vi "Amplifier Daemon.vi"(0 "Multiclamp Reference":i32, 1 "Signal":refnum<vi>, 2 "Gain":refnum<vi>, 3 "Autotune Gain":T4, 4 "Test Signal":T3, 5 "Error In":errorcluster, 6 "Capacitance Compensation":T5, 7 "Pipette Offset":T1, 9 "Holding Potential":T2, 11 "Reset":refnum<vi>, 13 "Exit":refnum<vi>) -> (19 "Error Out":errorcluster)   [LabVIEW 2012, in "MultiClamp 700B Controls.lvlib"]
uses:
  MultiClamp 700B Controls.lvlib
  AxMultiClampMsg/AxMultiClampMsg.lvlib
panel:
  out "Exit":bool
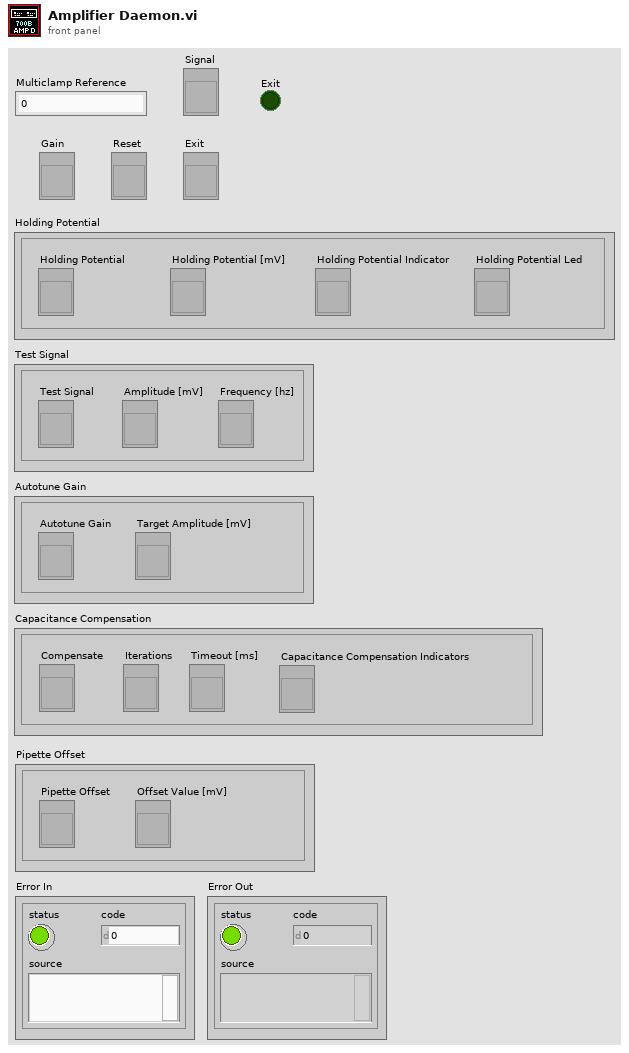
[diagram p1: front panel]
types:
  T1 = cluster{"Pipette Offset":refnum<vi>, "Offset Value [mV]":refnum<vi>}
  T2 = cluster{"Holding Potential [mV]":refnum<vi>, "Holding Potential":refnum<vi>, "Holding Potential Indicator":refnum<vi>, "Holding Potential Led":refnum<vi>}
  T3 = cluster{"Test Signal":refnum<vi>, "Amplitude [mV]":refnum<vi>, "Frequency [hz]":refnum<vi>}
  T4 = cluster{"Autotune Gain":refnum<vi>, "Target Amplitude [mV]":refnum<vi>}
  T5 = cluster{"Timeout [ms]":refnum<vi>, "Iterations":refnum<vi>, "Compensate":refnum<vi>, "Capacitance Compensation Indicators":refnum<vi>}
  T6 = cluster{"Cp Fast [pF]":dbl, "Cp Slow [pF]":dbl, "Tau Fast [um]":dbl, "Tau Slow [um]":dbl}
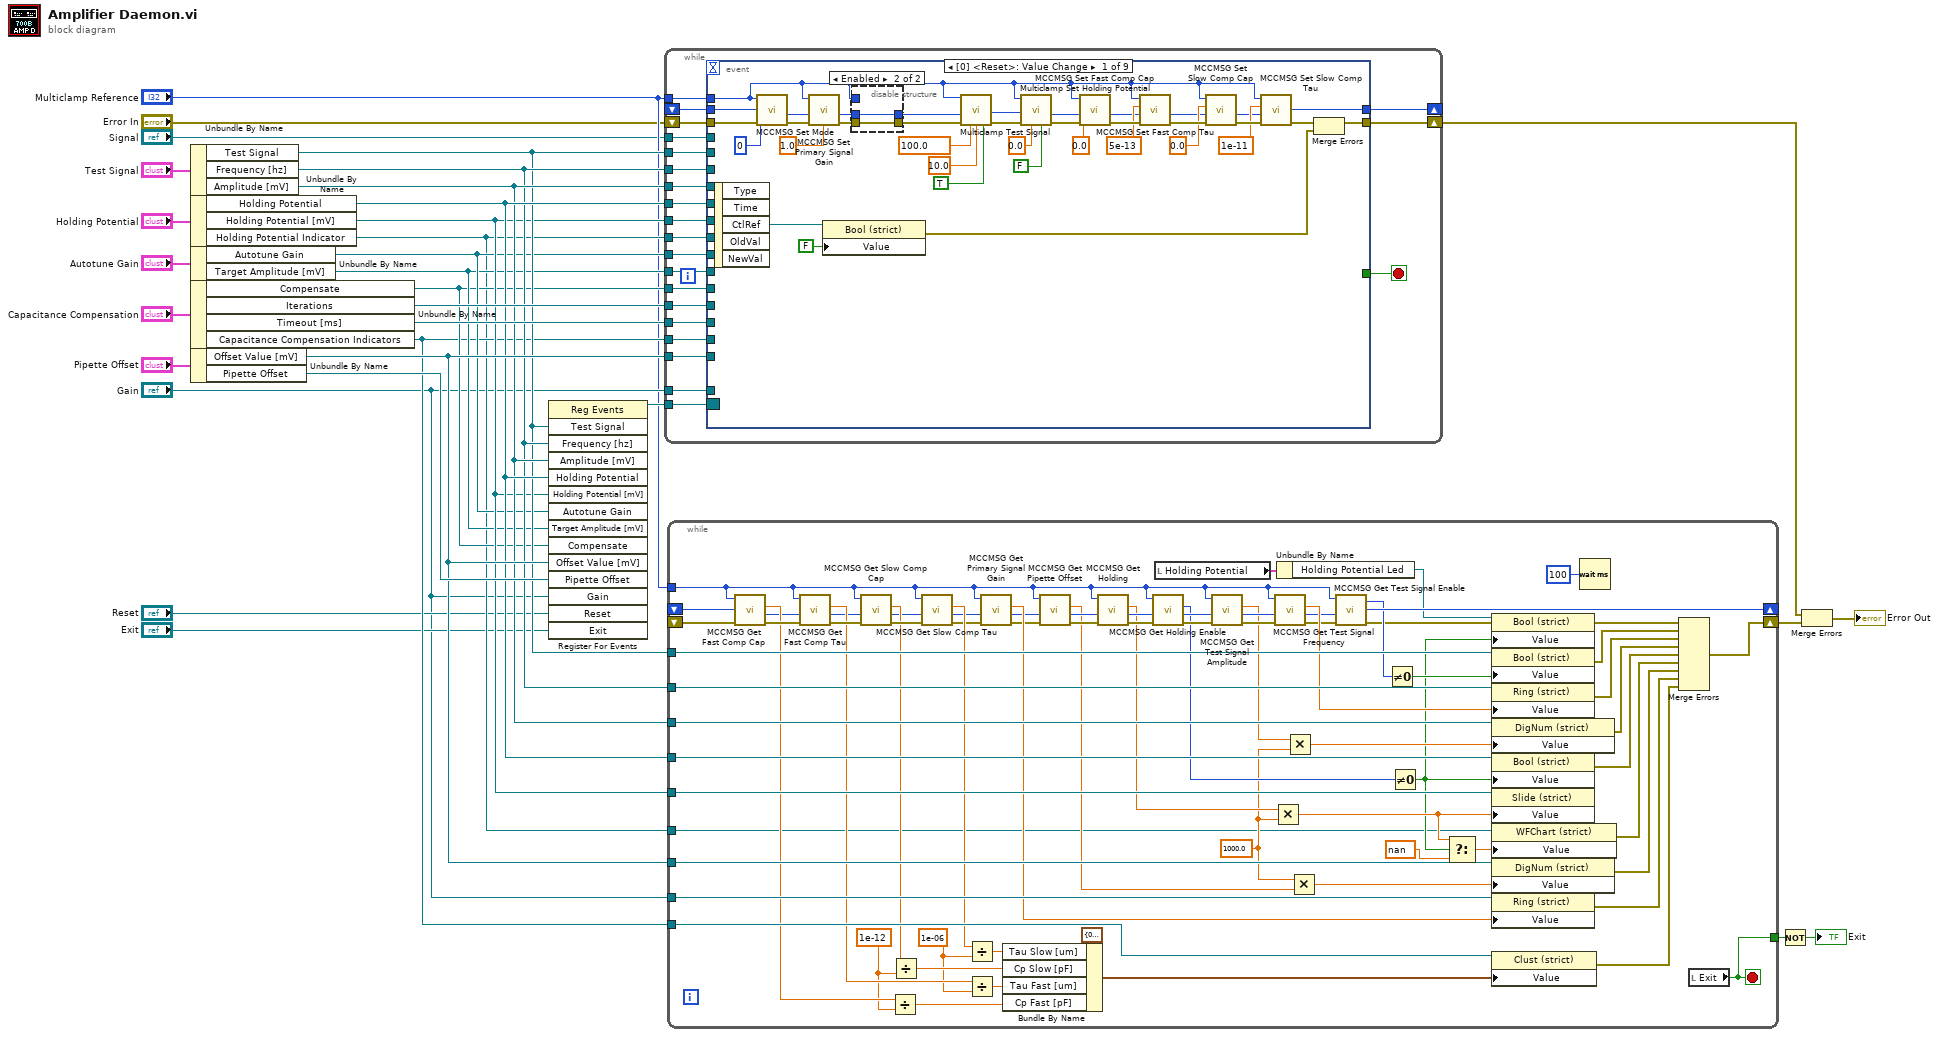
[diagram p0: block diagram]
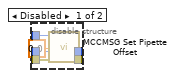
[diagram p2: hidden frame]
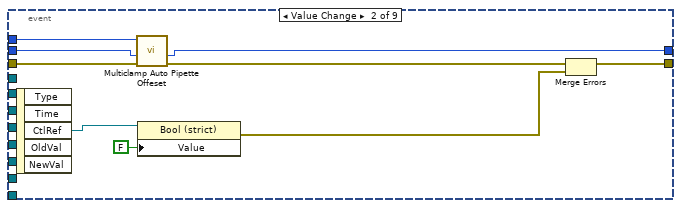
[diagram p3: hidden frame]
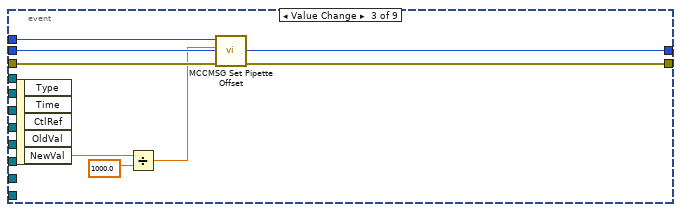
[diagram p4: hidden frame]
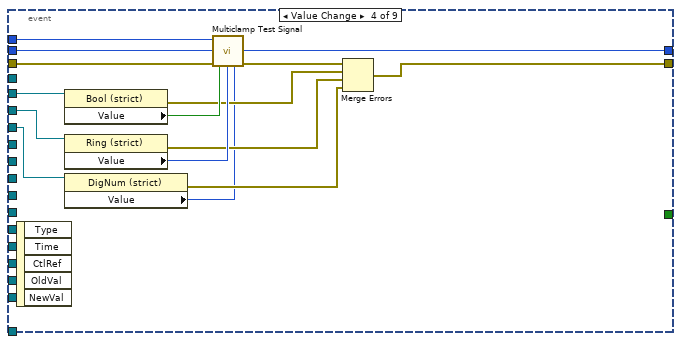
[diagram p5: hidden frame]
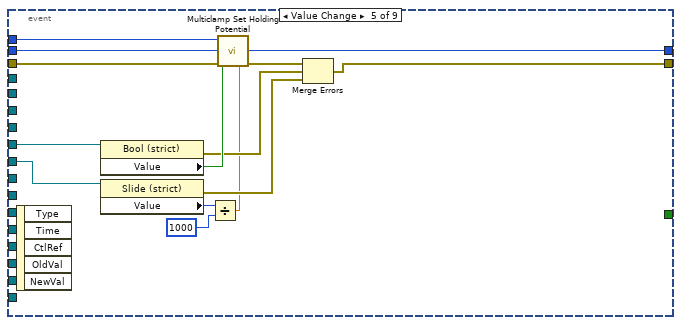
[diagram p6: hidden frame]
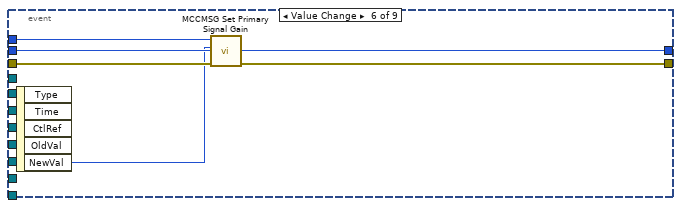
[diagram p7: hidden frame]
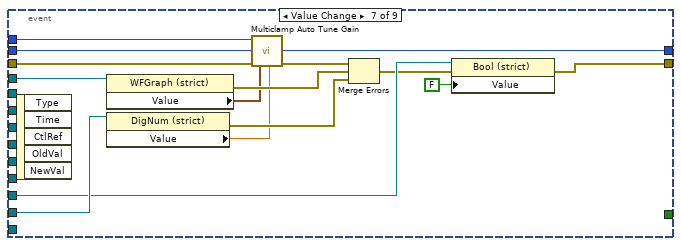
[diagram p8: hidden frame]
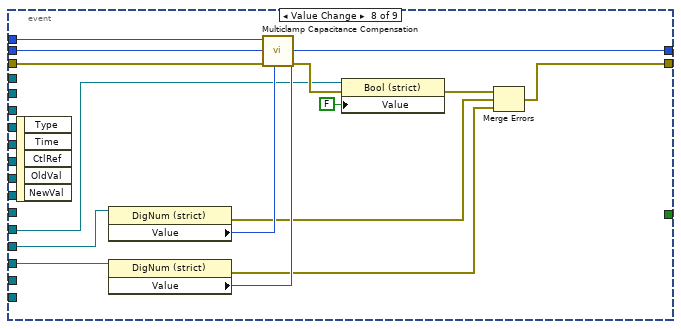
[diagram p9: hidden frame]
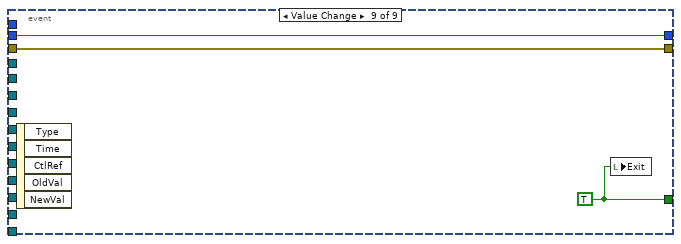
[diagram p10: hidden frame]
diagram:
  n1 = Unbundle By Name("Test Signal") -> ("Test Signal"=w23:refnum<vi>, "Frequency [hz]"=w24:refnum<vi>, "Amplitude [mV]"=w25:refnum<vi>)
  n2 = Unbundle By Name("Holding Potential") -> ("Holding Potential"=w26:refnum<vi>, "Holding Potential [mV]"=w22:refnum<vi>, "Holding Potential Indicator"=w17:refnum<vi>)
  n3 = Unbundle By Name("Autotune Gain") -> ("Autotune Gain"=w21:refnum<vi>, "Target Amplitude [mV]"=w20:refnum<vi>)
  n4 = Unbundle By Name("Capacitance Compensation") -> ("Compensate"=w19:refnum<vi>, "Iterations"=w30:refnum<vi>, "Timeout [ms]"=w29:refnum<vi>, "Capacitance Compensation Indicators"=w18:refnum<vi>)
  n5 = Unbundle By Name("Pipette Offset") -> ("Offset Value [mV]"=w27:refnum<vi>, "Pipette Offset"=w28:refnum<vi>)
  n6 = register-events(w23, w24, w25, w26, w22, w21, w20, w19, w27, w28, "Gain", "Reset", "Exit") -> (reference out=w31:refnum<event-registration>)  [unwired: 2 in, 1 out]
  n7 = while {
    tunnel: w31 -> [w53]
    tunnel: "Multiclamp Reference" -> [w52]
    tunnel: w24 -> [w51]
    tunnel: w25 -> [w50]
    tunnel: w23 -> [w49]
    tunnel: w26 -> [w48]
    tunnel: w22 -> [w47]
    tunnel: w20 -> [w46]
    tunnel: "Signal" -> [w45]
    tunnel: w30 -> [w44]
    tunnel: w29 -> [w43]
    tunnel: w21 -> [w42]
    tunnel: w19 -> [w41]
    shift-right: [w40] -> w15
    shift-left: "Error In" -> [w39]
    tunnel: w27 -> [w38]
    shift-right: [w36] -> _
    shift-left: _ -> [w37]
    tunnel: w18 -> [w34]
    tunnel: w17 -> [w33]
    tunnel: "Gain" -> [w32]
    stop <- w35 stop-if-true
    n8 = event shown="[0] <Reset>: Value Change" {
      selector: w53 -> [_ _ _ _ _ _ _ _ _]
      dyn-events: _ -> [_ _ _ _ _ _ _ _ _]
      timeout: _ -> [_ _ _ _ _ _ _ _ _]
      tunnel: w52 -> [w75 w106 w114 w129 w141 w148 w163 w179 _]
      tunnel: w51 -> [_ _ _ w128 _ _ _ _ _]
      tunnel: w50 -> [_ _ _ w116 _ _ _ _ _]
      tunnel: w49 -> [_ _ _ w126 _ _ _ _ _]
      tunnel: w48 -> [_ _ _ _ w143 _ _ _ _]
      tunnel: w47 -> [_ _ _ _ w142 _ _ _ _]
      tunnel: w46 -> [_ _ _ _ _ _ w164 _ _]
      tunnel: w45 -> [_ _ _ _ _ _ w162 _ _]
      tunnel: w44 -> [_ _ _ _ _ _ _ w176 _]
      tunnel: w43 -> [_ _ _ _ _ _ _ w177 _]
      tunnel: w42 -> [_ _ _ _ _ _ w161 _ _]
      tunnel: w41 -> [_ _ _ _ _ _ _ w166 _]
      tunnel: [w67 w100 w112 w119 w135 w147 w152 w172 w181] -> w40
      tunnel: w39 -> [w77 w104 w113 w124 w139 w149 w159 w174 w181]
      tunnel: w38 -> [_ _ _ _ _ _ _ _ _]
      tunnel: w37 -> [w64 w102 w111 w118 w134 w145 w156 w168 w182]
      tunnel: [w55 w101 w110 w117 w133 w146 w155 w167 w182] -> w36
      tunnel: [_ _ _ _ _ _ _ _ w180] -> w35
      tunnel: w34 -> [_ _ _ _ _ _ _ _ _]
      tunnel: w33 -> [_ _ _ _ _ _ _ _ _]
      tunnel: w32 -> [_ _ _ _ _ _ _ _ _]
      event Value Change {
        w73 = 100.0 items=["2 Hz"=2.0, "5 Hz"=5.0, "10 Hz"=10.0, "20 Hz"=20.0, "50 Hz"=50.0, "60 Hz"=60.0, "100 Hz"=100.0, "200 Hz"=200.0, "500 Hz"=500.0, "1000 Hz"=1000.0] ("Frequency")
        n9 = event-data() -> ("CtlRef"=w68:refnum<vi>)  [unwired: 1 in, 4 out]
        n10 = call "MCCMSG Set Mode.vi"("error in (no error)"=w77, "pnError"=w64, "uModeID"=u32 0, "hMCCmsg"=w75) -> ("error out"=w76:errorcluster, "pnError out"=w63:i32)  [unwired: 5 in, 1 out]
        n11 = call "MCCMSG Set Primary Signal Gain.vi"("error in (no error)"=w76, "pnError"=w63, "dGain"=1.0, "hMCCmsg"=w75) -> ("error out"=w89:errorcluster, "pnError out"=w62:i32)  [unwired: 5 in, 1 out]
        n12 = property class="Bool (strict)"(reference=w68, "Value"=FALSE) -> (error out=w65:errorcluster)  [unwired: 1 in, 1 out]
        n13 = disable-structure shown="Enabled" {
          disable-tunnel: w89 -> [w95 w97]
          disable-tunnel: [w94 w97] -> w80
          disable-tunnel: w75 -> [w93 _]
          disable-tunnel: w62 -> [w92 w96]
          disable-tunnel: [w91 w96] -> w61
          frame Disabled {
            n14 = call "MCCMSG Set Pipette Offset.vi"("error in (no error)"=w95, "pnError"=w92, "dPipetteOffset"=0.0, "hMCCmsg"=w93) -> ("error out"=w94:errorcluster, "pnError out"=w91:i32)  [unwired: 5 in, 1 out]
          }
          frame Enabled {
          }
        }
        n15 = call "Multiclamp Test Signal.vi"("Handler"=w75, "set"=TRUE, "pnErrorIn"=w61, "error in (no error)"=w80, "Frequency"=w73, "Amplitude [mV]"=10.0 ("Amplitude")) -> ("pnError out"=w60:i32, "error out"=w79:errorcluster)  [unwired: 7 in, 1 out]
        n16 = call "Multiclamp Set Holding Potential.vi"("On"=FALSE, "error in (no error)"=w79, "Voltage"=0.0, "pnError"=w60, "hMCCmsg"=w75) -> ("error out"=w78:errorcluster, "pnError out"=w56:i32)  [unwired: 4 in, 1 out]
        n17 = call "MCCMSG Set Fast Comp Cap.vi"("error in (no error)"=w78, "pnError"=w56, "dFastCompCap"=0.0, "hMCCmsg"=w75) -> ("error out"=w88:errorcluster, "pnError out"=w57:i32)  [unwired: 5 in, 1 out]
        n18 = call "MCCMSG Set Fast Comp Tau.vi"("error in (no error)"=w88, "pnError"=w57, "dFastCompTau"=5e-13, "hMCCmsg"=w75) -> ("error out"=w87:errorcluster, "pnError out"=w58:i32)  [unwired: 5 in, 1 out]
        n19 = call "MCCMSG Set Slow Comp Cap.vi"("error in (no error)"=w87, "pnError"=w58, "dSlowCompCap"=0.0, "hMCCmsg"=w75) -> ("error out"=w86:errorcluster, "pnError out"=w59:i32)  [unwired: 5 in, 1 out]
        n20 = call "MCCMSG Set Slow Comp Tau.vi"("error in (no error)"=w86, "pnError"=w59, "dSlowCompTau"=1e-11, "hMCCmsg"=w75) -> ("error out"=w66:errorcluster, "pnError out"=w55:i32)  [unwired: 5 in, 1 out]
        n21 = Merge Errors(w66, w65) -> (w67:errorcluster)
      }
      event Value Change {
        n22 = event-data() -> ("CtlRef"=w105:refnum<vi>)  [unwired: 1 in, 4 out]
        n23 = call "Multiclamp Auto Pipette Offeset.vi"("error in (no error)"=w104, "pnError"=w102, "hMCCmsg"=w106) -> ("error out"=w103:errorcluster, "pnError out"=w101:i32)  [unwired: 6 in, 1 out]
        n24 = property class="Bool (strict)"(reference=w105, "Value"=FALSE) -> (error out=w99:errorcluster)  [unwired: 1 in, 1 out]
        n25 = Merge Errors(w103, w99) -> (w100:errorcluster)
      }
      event Value Change {
        n26 = event-data() -> ("NewVal"=w109:dbl)  [unwired: 1 in, 4 out]
        n27 = Divide(x=w109, y=1000.0) -> (x/y=w108:dbl)
        n28 = call "MCCMSG Set Pipette Offset.vi"("error in (no error)"=w113, "pnError"=w111, "dPipetteOffset"=w108, "hMCCmsg"=w114) -> ("error out"=w112:errorcluster, "pnError out"=w110:i32)  [unwired: 5 in, 1 out]
      }
      event Value Change {
        n29 = event-data() -> ()  [unwired: 1 in, 5 out]
        n30 = property class="Bool (strict)"(reference=w126) -> (error out=w122:errorcluster, "Value"=w127:bool)  [unwired: 1 in, 1 out]
        n31 = property class="Ring (strict)"(reference=w128) -> (error out=w121:errorcluster, "Value"=w125:u16)  [unwired: 1 in, 1 out]
        n32 = property class="DigNum (strict)"(reference=w116) -> (error out=w120:errorcluster, "Value"=w115:i32)  [unwired: 1 in, 1 out]
        n33 = call "Multiclamp Test Signal.vi"("Handler"=w129, "set"=w127, "pnErrorIn"=w118, "error in (no error)"=w124, "Frequency"=w125, "Amplitude [mV]"=w115) -> ("pnError out"=w117:i32, "error out"=w123:errorcluster)  [unwired: 7 in, 1 out]
        n34 = Merge Errors(w123, w122, w121, w120) -> (w119:errorcluster)
      }
      event Value Change {
        n35 = event-data() -> ()  [unwired: 1 in, 5 out]
        n36 = property class="Bool (strict)"(reference=w143) -> (error out=w137:errorcluster, "Value"=w140:bool)  [unwired: 1 in, 1 out]
        n37 = property class="Slide (strict)"(reference=w142) -> (error out=w136:errorcluster, "Value"=w132:i32)  [unwired: 1 in, 1 out]
        n38 = Divide(x=w132, y=1000) -> (x/y=w131:dbl)
        n39 = call "Multiclamp Set Holding Potential.vi"("On"=w140, "error in (no error)"=w139, "Voltage"=w131, "pnError"=w134, "hMCCmsg"=w141) -> ("error out"=w138:errorcluster, "pnError out"=w133:i32)  [unwired: 4 in, 1 out]
        n40 = Merge Errors(w138, w137, w136) -> (w135:errorcluster)
      }
      event Value Change {
        n41 = event-data() -> ("NewVal"=w144:u16)  [unwired: 1 in, 4 out]
        n42 = call "MCCMSG Set Primary Signal Gain.vi"("error in (no error)"=w149, "pnError"=w145, "dGain"=w144, "hMCCmsg"=w148) -> ("error out"=w147:errorcluster, "pnError out"=w146:i32)  [unwired: 5 in, 1 out]
      }
      event Value Change {
        n43 = event-data() -> ()  [unwired: 1 in, 5 out]
        n44 = property class="WFGraph (strict)"(reference=w162) -> (error out=w157:errorcluster, "Value"=w151:waveform(dbl))  [unwired: 1 in, 1 out]
        n45 = property class="DigNum (strict)"(reference=w164) -> (error out=w154:errorcluster, "Value"=w150:dbl)  [unwired: 1 in, 1 out]
        n46 = call "Multiclamp Auto Tune Gain.vi"("Target Delta pp"=w150, "error in (no error)"=w159, "pnError"=w156, "Multiclamp Reference"=w163, "Test Signal"=w151) -> ("error out"=w158:errorcluster, "pnError out"=w155:i32)  [unwired: 3 in, 2 out]
        n47 = Merge Errors(w158, w157, w154) -> (w153:errorcluster)
        n48 = property class="Bool (strict)"(reference=w161, error in=w153, "Value"=FALSE) -> (error out=w152:errorcluster)  [unwired: 1 out]
      }
      event Value Change {
        n49 = event-data() -> ()  [unwired: 1 in, 5 out]
        n50 = property class="DigNum (strict)"(reference=w176) -> (error out=w170:errorcluster, "Value"=w175:i32)  [unwired: 1 in, 1 out]
        n51 = property class="DigNum (strict)"(reference=w177) -> (error out=w169:errorcluster, "Value"=w178:u32)  [unwired: 1 in, 1 out]
        n52 = call "Multiclamp Capacitance Compensation.vi"("#i"=w175, "error in (no error)"=w174, "Timeout [ms]"=w178, "pnError"=w168, "hMCCmsg"=w179) -> ("error out"=w173:errorcluster, "pnError out"=w167:i32)  [unwired: 4 in, 1 out]
        n53 = property class="Bool (strict)"(reference=w166, error in=w173, "Value"=FALSE) -> (error out=w171:errorcluster)  [unwired: 1 out]
        n54 = Merge Errors(w171, w170, w169) -> (w172:errorcluster)
      }
      event Value Change {
        w180 = TRUE ("NewVal")
        n55 = event-data() -> ()  [unwired: 1 in, 5 out]
        n56 = local write "Exit"(w180) -> ()
      }
    }
  }
  n57 = while {
    shift-right: [w257] -> w16
    shift-left: _ -> [w256]
    shift-right: [w254] -> _
    shift-left: _ -> [w255]
    tunnel: w18 -> [w253]
    tunnel: "Gain" -> [w252]
    tunnel: w27 -> [w251]
    tunnel: w17 -> [w187]
    tunnel: w26 -> [w250]
    tunnel: w25 -> [w249]
    tunnel: w24 -> [w248]
    tunnel: w23 -> [w247]
    tunnel: "Multiclamp Reference" -> [w246]
    tunnel: w22 -> [w245]
    tunnel: [w194] -> w2
    stop <- w194 stop-if-true
    w195 = 1000.0 ("y")
    w232 = 1e-06 ("y")
    w233 = 1e-12 ("y")
    n58 = call "MCCMSG Get Fast Comp Cap.vi"("error in (no error)"=w256, "pnError"=w255, "hMCCmsg"=w246) -> ("error out"=w242:errorcluster, "pnError out"=w204:i32, "pdFastCompCap out"=w238:dbl)  [unwired: 5 in, 1 out]
    n59 = call "MCCMSG Get Fast Comp Tau.vi"("error in (no error)"=w242, "pnError"=w204, "hMCCmsg"=w246) -> ("error out"=w244:errorcluster, "pnError out"=w205:i32, "pdFastCompTau out"=w234:dbl)  [unwired: 5 in, 1 out]
    n60 = call "MCCMSG Get Slow Comp Cap.vi"("error in (no error)"=w244, "pnError"=w205, "hMCCmsg"=w246) -> ("error out"=w243:errorcluster, "pnError out"=w206:i32, "pdSlowCompCap out"=w241:dbl)  [unwired: 5 in, 1 out]
    n61 = Divide(x=w238, y=w233) -> (x/y=w239:dbl)
    n62 = Divide(x=w241, y=w233) -> (x/y=w240:dbl)
    n63 = call "MCCMSG Get Slow Comp Tau.vi"("error in (no error)"=w243, "pnError"=w206, "hMCCmsg"=w246) -> ("error out"=w214:errorcluster, "pnError out"=w207:i32, "pdSlowCompTau out"=w236:dbl)  [unwired: 5 in, 1 out]
    n64 = Divide(x=w236, y=w232) -> (x/y=w237:dbl)
    n65 = Divide(x=w234, y=w232) -> (x/y=w235:dbl)
    n66 = call "MCCMSG Get Primary Signal Gain.vi"("error in (no error)"=w214, "pnError"=w207, "hMCCmsg"=w246) -> ("error out"=w215:errorcluster, "pnError out"=w208:i32, "pdGain out"=w225:dbl)  [unwired: 5 in, 1 out]
    n67 = Bundle By Name(cluster=T6 {"Cp Fast [pF]"=0.0, "Cp Slow [pF]"=0.0, "Tau Fast [um]"=0.0, "Tau Slow [um]"=0.0} ("Dummy"), "Tau Slow [um]"=w237, "Cp Slow [pF]"=w240, "Tau Fast [um]"=w235, "Cp Fast [pF]"=w239) -> (w226:T6)
    n68 = call "MCCMSG Get Pipette Offset.vi"("error in (no error)"=w215, "pnError"=w208, "hMCCmsg"=w246) -> ("error out"=w216:errorcluster, "pnError out"=w209:i32, "pdPipetteOffset out"=w199:dbl)  [unwired: 5 in, 1 out]
    n69 = call "MCCMSG Get Holding.vi"("error in (no error)"=w216, "pnError"=w209, "hMCCmsg"=w246) -> ("error out"=w224:errorcluster, "pnError out"=w210:i32, "pdHolding out"=w198:dbl)  [unwired: 5 in, 1 out]
    n70 = call "MCCMSG Get Holding Enable.vi"("error in (no error)"=w224, "pnError"=w210, "hMCCmsg"=w246) -> ("error out"=w223:errorcluster, "pnError out"=w211:i32, "pbEnable out"=w203:i32)  [unwired: 5 in, 1 out]
    n71 = local read "Holding Potential"() -> (w192:T2)
    n72 = call "MCCMSG Get Test Signal Amplitude.vi"("error in (no error)"=w223, "pnError"=w211, "hMCCmsg"=w246) -> ("error out"=w222:errorcluster, "pnError out"=w212:i32, "pdAmplitude out"=w202:dbl)  [unwired: 5 in, 1 out]
    n73 = Multiply(x=w198, y=w195) -> (x*y=w196:dbl)
    n74 = call "MCCMSG Get Test Signal Frequency.vi"("error in (no error)"=w222, "pnError"=w212, "hMCCmsg"=w246) -> ("error out"=w221:errorcluster, "pnError out"=w213:i32, "pdFrequency out"=w228:dbl)  [unwired: 5 in, 1 out]
    n75 = Unbundle By Name(w192) -> ("Holding Potential Led"=w191:refnum<vi>)
    n76 = Multiply(x=w202, y=w195) -> (x*y=w201:dbl)
    n77 = Multiply(x=w195, y=w199) -> (x*y=w200:dbl)
    n78 = call "MCCMSG Get Test Signal Enable.vi"("error in (no error)"=w221, "pnError"=w213, "hMCCmsg"=w246) -> ("error out"=w189:errorcluster, "pnError out"=w254:i32, "pbEnable out"=w229:i32)  [unwired: 5 in, 1 out]
    n79 = Not Equal To 0?(x=w229) -> (x != 0?=w230:bool)
    n80 = Not Equal To 0?(x=w203) -> (x != 0?=w188:bool)
    n81 = Select(t=w196, s=w188, f=nan) -> (s? t:f=w197:dbl)
    n82 = property class="Bool (strict)"(reference=w191, error in=w189, "Value"=w188) -> (error out=w190:errorcluster)  [unwired: 1 out]
    n83 = property class="Bool (strict)"(reference=w247, "Value"=w230) -> (error out=w220:errorcluster)  [unwired: 1 in, 1 out]
    n84 = property class="Ring (strict)"(reference=w248, "Value"=w228) -> (error out=w219:errorcluster)  [unwired: 1 in, 1 out]
    n85 = property class="DigNum (strict)"(reference=w249, "Value"=w201) -> (error out=w218:errorcluster)  [unwired: 1 in, 1 out]
    n86 = property class="Bool (strict)"(reference=w250, "Value"=w188) -> (error out=w217:errorcluster)  [unwired: 1 in, 1 out]
    n87 = property class="Slide (strict)"(reference=w245, "Value"=w196) -> ()  [unwired: 1 in, 2 out]
    n88 = property class="WFChart (strict)"(reference=w187, "Value"=w197) -> (error out=w186:errorcluster)  [unwired: 1 in, 1 out]
    n89 = property class="DigNum (strict)"(reference=w251, "Value"=w200) -> (error out=w185:errorcluster)  [unwired: 1 in, 1 out]
    n90 = property class="Ring (strict)"(reference=w252, "Value"=w225) -> (error out=w184:errorcluster)  [unwired: 1 in, 1 out]
    n91 = property class="Clust (strict)"(reference=w253, "Value"=w226) -> (error out=w183:errorcluster)  [unwired: 1 in, 1 out]
    n92 = Wait (ms)(milliseconds to wait=u32 100) -> ()  [unwired: 1 out]
    n93 = Merge Errors(w190, w220, w219, w218, w217, w186, w185, w184, w183) -> (w257:errorcluster)
    n94 = local read "Exit"() -> (w194:bool)
  }
  n95 = Not(x=w2) -> (.not. x?=→"Exit":bool)
  n96 = Merge Errors(w15, w16) -> (→"Error Out":errorcluster)
